vi "test_clock_routing.vi"(8 "error in (no error)":errorcluster) -> (0 "error out":errorcluster)   [LabVIEW 2012]
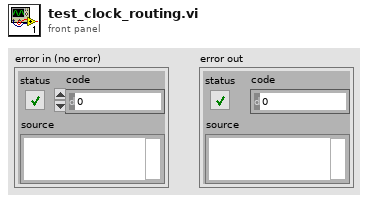
[diagram p1: front panel]
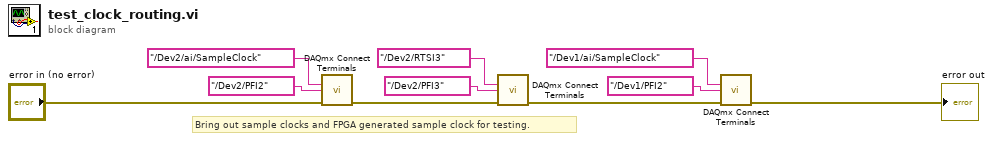
[diagram p0: block diagram]
diagram:
  # "Bring out sample clocks and FPGA generated sample clock for testing."
  n1 = call <vilib>:"DAQmx Connect Terminals.vi"("source terminal"=tag "/Dev2/ai/SampleClock", "destination terminal"=tag "/Dev2/PFI2", "error in"="error in (no error)") -> ("error out"=w5:errorcluster)  [unwired: 12 in]
  n2 = call <vilib>:"DAQmx Connect Terminals.vi"("source terminal"=tag "/Dev2/RTSI3", "destination terminal"=tag "/Dev2/PFI3", "error in"=w5) -> ("error out"=w8:errorcluster)  [unwired: 12 in]
  n3 = call <vilib>:"DAQmx Connect Terminals.vi"("source terminal"=tag "/Dev1/ai/SampleClock", "destination terminal"=tag "/Dev1/PFI2", "error in"=w8) -> ("error out"=→"error out":errorcluster)  [unwired: 12 in]
